vi "strip positioning.vi"(1 "result string 2":string) -> (0 "result string":string)   [LabVIEW 2018]
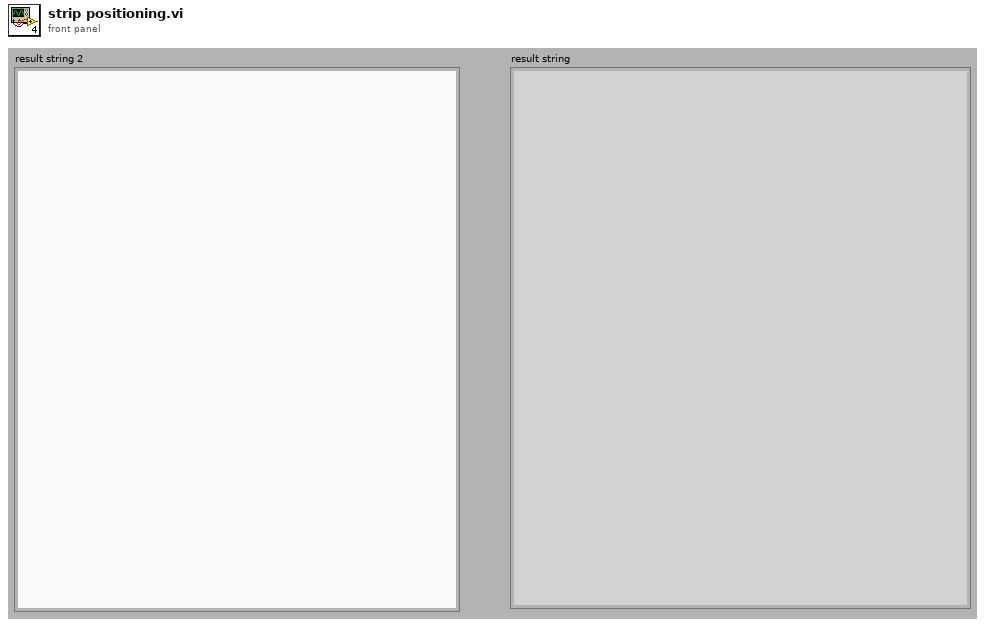
[diagram p1: front panel]
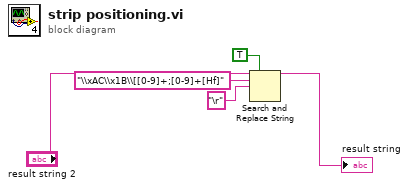
[diagram p0: block diagram]
diagram:
  n1 = Search and Replace String(replace all?=TRUE ("replace all? (F)"), input string="result string 2", search string="\\xAC\\x1B\\[[0-9]+;[0-9]+[Hf]", replace string="\r" ("search string")) -> (result string=→"result string":string)  [unwired: 4 in, 3 out]
